vi "circle fit data.vi"(2 "y偏移(b)":dbl, 3 "x偏移(a)":dbl, 4 "半径":dbl, 5 "采样":i32) -> (0 "Y":dbl[](array[numeric]), 1 "X":dbl[](array[numeric]))   [LabVIEW 2016]
doc: "拟合数据－圆"
uses:
  <vilib>/Analysis/1siggen.llb/Ramp Pattern by Samples.vi
  <vilib>/Analysis/NI_AALBase.lvlib
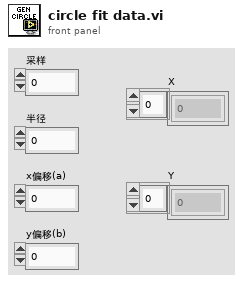
[diagram p1: front panel]
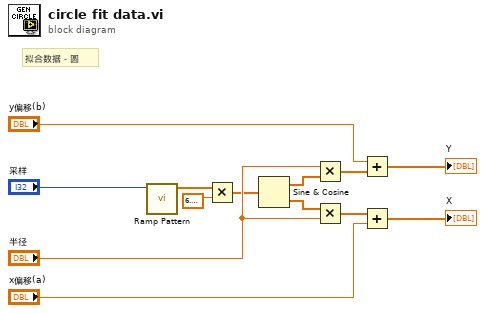
[diagram p0: block diagram]
diagram:
  # "拟合数据－圆"
  n1 = call-poly <vilib>:"Ramp Pattern.vi"("samples"="采样") -> ("Ramp Pattern"=w3:dbl[])  [unwired: 9 in, 1 out]
  n2 = Multiply(x=w3, y=6.283185307179586) -> (x*y=w5:dbl[])
  n3 = Sine & Cosine(0:w5) -> (1:w8:dbl[], 2:w6:dbl[])
  n4 = Multiply(x="半径", y=w8) -> (x*y=w1:dbl[])
  n5 = Multiply(x=w6, y="半径") -> (x*y=w9:dbl[])
  n6 = Add(x="y偏移(b)", y=w1) -> (x+y=→"Y":dbl[])
  n7 = Add(x=w9, y="x偏移(a)") -> (x+y=→"X":dbl[])
